vi "Command Line.vi"(0 "COM Port in":refnum<visa-resource-name>, 1 "Command":string, 2 "error in":errorcluster) -> (3 "COM Port out":refnum<visa-resource-name>, 4 "OK":bool, 5 "Return":string, 6 "error out":errorcluster)   [LabVIEW 2013]
doc: "This VI sends a written command to the device and displays the answer."
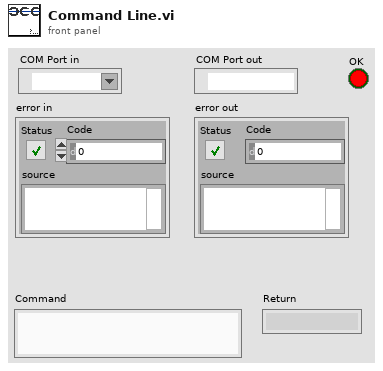
[diagram p1: front panel]
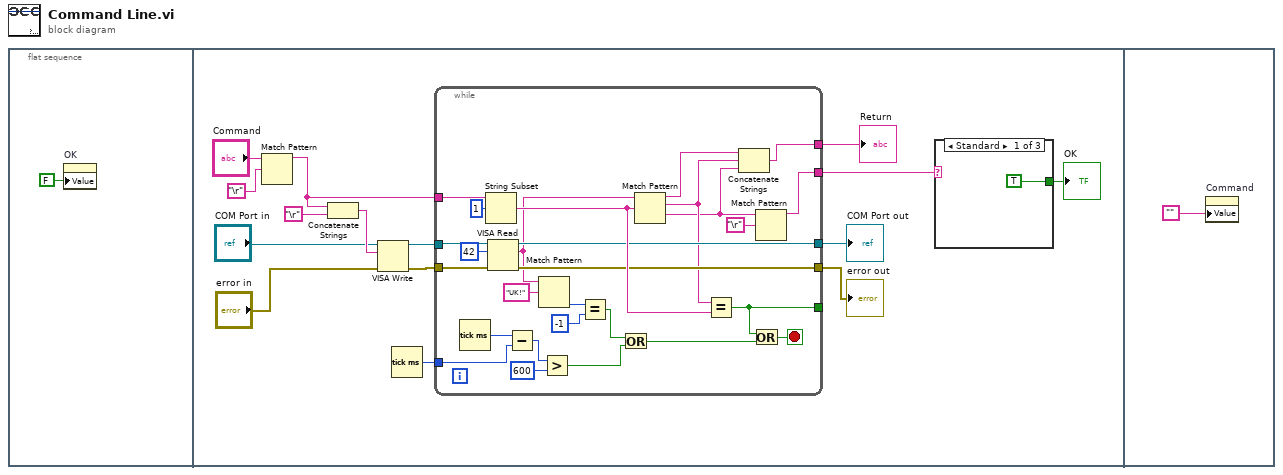
[diagram p0: block diagram]
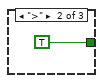
[diagram p2: hidden frame]
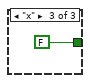
[diagram p3: hidden frame]
diagram:
  n1 = flat-sequence {
    frame #0 {
      n2 = property on="OK" class="Bool. (strikt)"("Value"=FALSE ("OK")) -> ()  [unwired: 2 in, 2 out]
    }
    frame #1 {
      n3 = Match Pattern(string="Command", regular expression="\r") -> (before substring=w3:string)  [unwired: 1 in, 3 out]
      n4 = Concatenate Strings(w3, "\r") -> (w14:string)
      n5 = VISA Write(VISA resource name="COM Port in", write buffer=w14, error in (no error)="error in") -> (VISA resource name out=w12:refnum<visa-resource-name>, error out=w11:errorcluster)  [unwired: 1 out]
      n6 = Tick Count (ms)() -> (millisecond timer value=w10:u32)
      n7 = while {
        tunnel: [w43] -> w16
        tunnel: [w42] -> w15
        tunnel: [w41] -> w9
        tunnel: [w38] -> _
        tunnel: w12 -> [w28]
        tunnel: w11 -> [w40]
        tunnel: w3 -> [w39]
        tunnel: w10 -> [w35]
        tunnel: [w30] -> w6
        stop <- w37 stop-if-true
        n8 = Tick Count (ms)() -> (millisecond timer value=w36:u32)
        n9 = String Subset(string=w39, offset (0)=1 ("Offset (0)")) -> (substring=w44:string)  [unwired: 1 in]
        n10 = VISA Read(VISA resource name=w28, byte count=u32 42 ("Byte-Anzahl"), error in (no error)=w40) -> (VISA resource name out=w43:refnum<visa-resource-name>, read buffer=w24:string, error out=w42:errorcluster)  [unwired: 1 out]
        n11 = Subtract(x=w36, y=w35) -> (x-y=w34:u32)
        n12 = Match Pattern(string=w24, regular expression="UK!" ("Regulärer Ausdruck")) -> (offset past match=w22:i32)  [unwired: 1 in, 3 out]
        n13 = Greater?(x=w34, y=u32 600) -> (0:w26:bool)
        n14 = Equal?(x=w22, y=-1) -> (x = y?=w20:bool)
        n15 = Or(x=w20, y=w26) -> (x .or. y?=w25:bool)
        n16 = Match Pattern(string=w24, regular expression=w44) -> (before substring=w32:string, match substring=w31:string, after substring=w29:string)  [unwired: 1 in, 1 out]
        n17 = Equal?(x=w31, y=w44) -> (x = y?=w38:bool)
        n18 = Concatenate Strings(w32, w31, w29) -> (w30:string)
        n19 = Or(x=w38, y=w25) -> (x .or. y?=w37:bool)
        n20 = Match Pattern(string=w29, regular expression="\r") -> (before substring=w41:string)  [unwired: 1 in, 3 out]
      }
      "COM Port out" <- w16
      "error out" <- w15
      "Return" <- w6
      n21 = case shown="Standard" w9 {
        tunnel: [TRUE TRUE FALSE] -> w8
        frame Default {
        }
        frame ">" {
        }
        frame "x" {
        }
      }
      "OK" <- w8
    }
    frame #2 {
      n22 = property on="Command" class="Str"("Value"="") -> ()  [unwired: 2 in, 2 out]
    }
  }
